vi "Save DAC Configuration.vi"(8 "error in":errorcluster, 10 "Config File refnum in":T1, 11 "DAC ADV in":refnum<class "DAC ADV.lvclass">) -> (0 "error out":errorcluster, 2 "Config File refnum out":T1, 3 "DAC ADV out":refnum<class "DAC ADV.lvclass">)   [LabVIEW 2019, in "DAC.lvlib" / "DAC ADV.lvclass"]
uses:
  DAC ADV.lvclass
  C:/Users/krio/Documents/LV_Projects/test-stand/App/DAC/DAC.lvclass
  <vilib>/Utility/config.llb/Config Data RefNum.ctl
  DAC.lvclass/DAC.ctl
  DAC ADV.lvclass/DAC ADV.ctl
  <vilib>/Utility/config.llb/Write Key (String).vi
  <vilib>/Utility/config.llb/Write Key (Double).vi
  DAC.lvclass
  <vilib>/Utility/config.llb/NI_LVConfig.lvlib
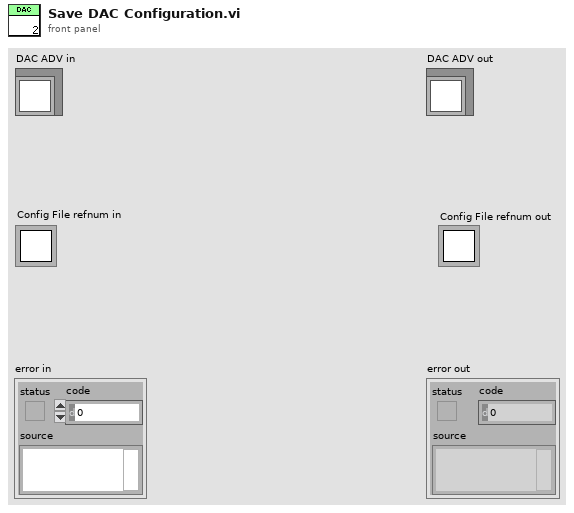
[diagram p1: front panel]
types:
  T1 = typedef "NI_LVConfig.lvlib/Config Data RefNum.ctl" = refnum<k1>
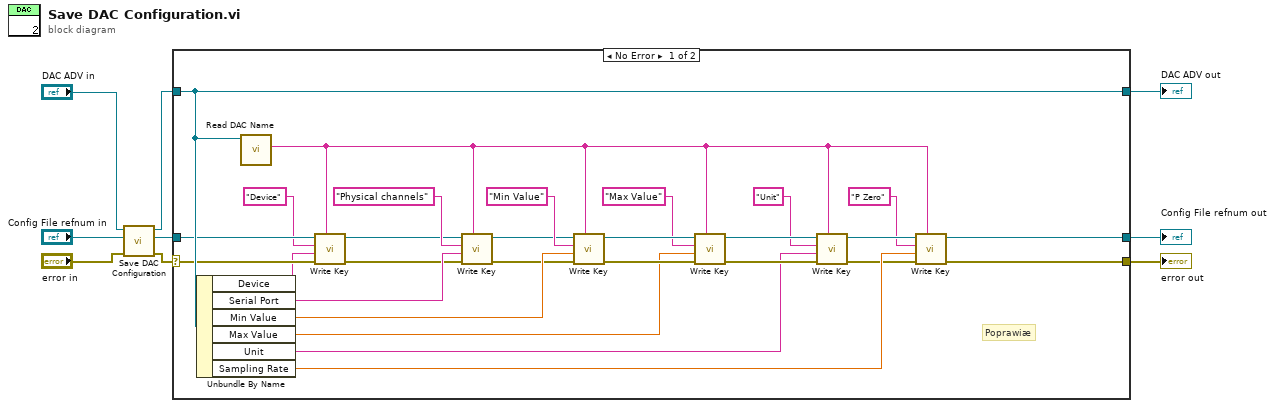
[diagram p0: block diagram]
diagram:
  n1 = call-parent "Save DAC Configuration.vi"("error in"="error in", "Config File refnum in"="Config File refnum in", "DAC in"="DAC ADV in") -> ("error out"=w4:errorcluster, "Config File refnum out"=w5:T1, "DAC out"=w6:refnum<class "DAC ADV.lvclass">)  [unwired: 6 in]
  n2 = case shown="No Error" w4 {
    selector: w4 -> [w20 w40]
    tunnel: [w10 w40] -> w1
    tunnel: [w26 w39] -> w3
    tunnel: w6 -> [w26 w39]
    tunnel: w5 -> [w21 w38]
    tunnel: [w15 w38] -> w2
    frame No Error {
      # "Poprawiæ"
      n3 = Unbundle By Name(w26) -> ("Device"=w16:string, "Serial Port"=w22:string, "Min Value"=w29:dbl, "Max Value"=w28:dbl, "Unit"=w27:string, "Sampling Rate"=w12:dbl)
      n4 = call "Read DAC Name.vi"("DAC in"=w26) -> ("DAC Name"=w14:string)  [unwired: 8 in, 2 out]
      n5 = call-poly <vilib>:"Write Key.vi"("section"=w14, "error in (no error)"=w20, "value"=w16, "key"="Device", "refnum"=w21) -> ("error out"=w18:errorcluster, "refnum out"=w19:T1)  [unwired: 4 in, 1 out]
      n6 = call-poly <vilib>:"Write Key.vi"("section"=w14, "error in (no error)"=w18, "value"=w22, "key"="Physical channels", "refnum"=w19) -> ("error out"=w24:errorcluster, "refnum out"=w25:T1)  [unwired: 4 in, 1 out]
      n7 = call-poly <vilib>:"Write Key.vi"("section"=w14, "error in (no error)"=w24, "value"=w29, "key"="Min Value", "refnum"=w25) -> ("error out"=w35:errorcluster, "refnum out"=w37:T1)  [unwired: 4 in, 1 out]
      n8 = call-poly <vilib>:"Write Key.vi"("section"=w14, "error in (no error)"=w35, "value"=w28, "key"="Max Value", "refnum"=w37) -> ("error out"=w34:errorcluster, "refnum out"=w36:T1)  [unwired: 4 in, 1 out]
      n9 = call-poly <vilib>:"Write Key.vi"("section"=w14, "error in (no error)"=w34, "value"=w27, "key"="Unit", "refnum"=w36) -> ("error out"=w11:errorcluster, "refnum out"=w30:T1)  [unwired: 4 in, 1 out]
      n10 = call-poly <vilib>:"Write Key.vi"("section"=w14, "error in (no error)"=w11, "value"=w12, "key"="P Zero", "refnum"=w30) -> ("error out"=w10:errorcluster, "refnum out"=w15:T1)  [unwired: 4 in, 1 out]
    }
    frame Error {
    }
  }
  "error out" <- w1
  "DAC ADV out" <- w3
  "Config File refnum out" <- w2
